vi "test_Open TCP connection using Clear Error node.vi"(8 "error in (no error)":errorcluster, 11 "TestCase in":refnum<class "Ethernet Protocol Tests.lvclass">) -> (0 "error out":errorcluster, 3 "TestCase out":refnum<class "Ethernet Protocol Tests.lvclass">)   [LabVIEW 2019, in "Ethernet Protocol Tests.lvclass"]
uses:
  Ethernet Protocol Tests.lvclass
  TCP/TCP.lvclass
  TCP/TCP.lvclass/TCP.ctl
  Constants.vi
  <vilib>/addons/_JKI Toolkits/VI Tester/TestCase.llb/TestCase.lvclass
  C:/Program Files (x86)/National Instruments/LabVIEW 2019/vi.lib/addons/_JKI Toolkits/VI Tester/TestCase.llb/TestCase.lvclass
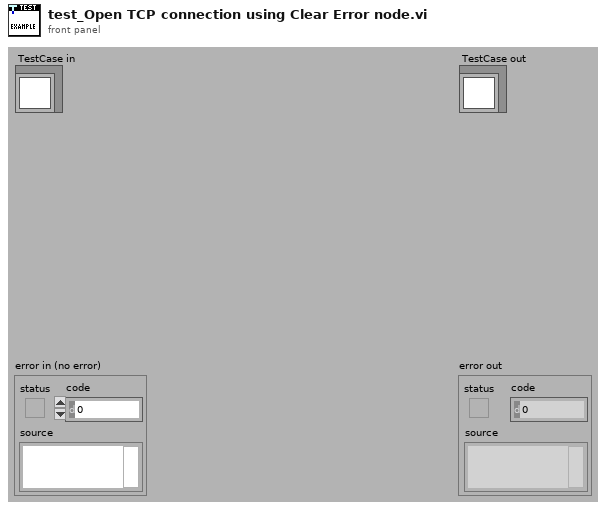
[diagram p1: front panel]
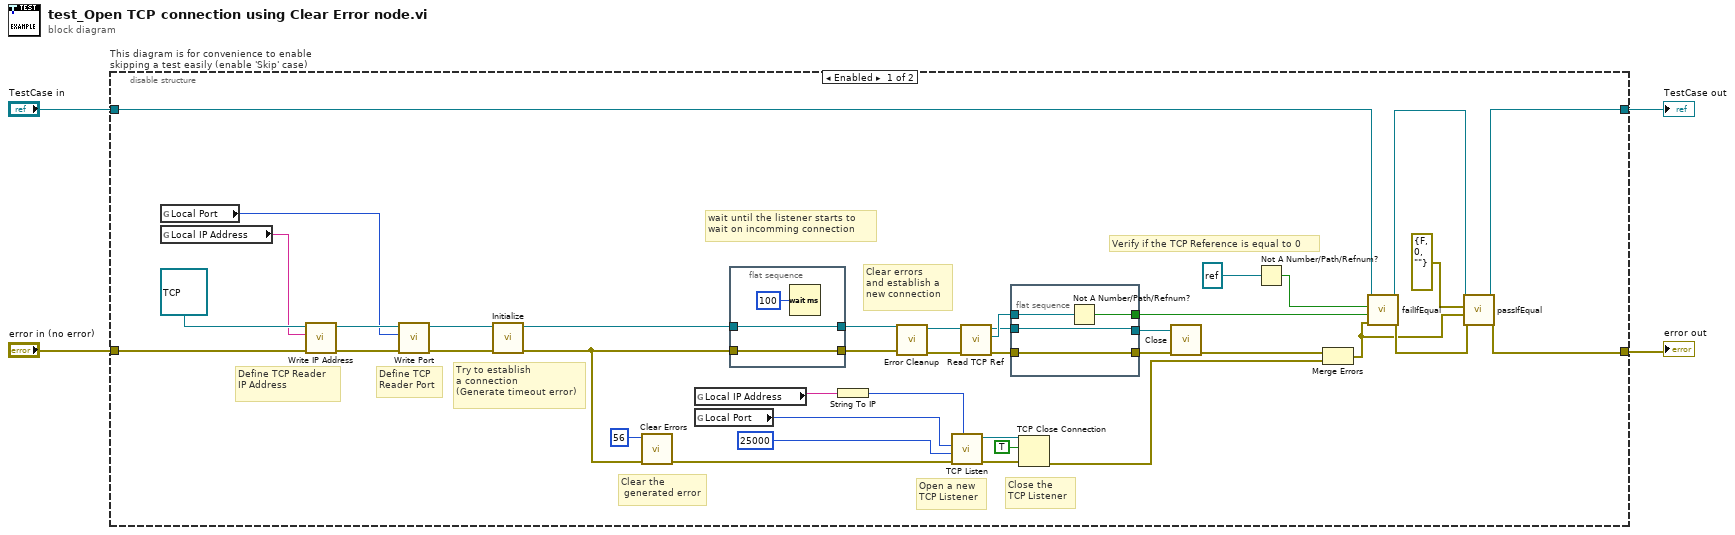
[diagram p0: block diagram]
diagram:
  n1 = disable-structure "This diagram is for convenience to enable skipping a test easily (enable 'Skip' case)" shown="Enabled" {
    disable-tunnel: "TestCase in" -> [w44 w55]
    disable-tunnel: [w12 w53] -> w1
    disable-tunnel: [w11 w54] -> w3
    disable-tunnel: "error in (no error)" -> [w40 w52]
    frame Enabled {
      # "Verify if the TCP Reference is equal to 0"
      # "Clear the\n generated error"
      # "Close the \nTCP Listener"
      # "Open a new \nTCP Listener"
      # "Clear errors \nand establish a \nnew connection"
      # "Try to establish \na connection\n(Generate timeout error)"
      # "wait until the listener starts to\nwait on incomming connection"
      # "Define TCP \nReader Port"
      # "Define TCP Reader \nIP Address"
      n2 = global read "Constants.vi" "Local Port"() -> (w19:u16)
      n3 = global read "Constants.vi" "Local IP Address"() -> (w20:string)
      n4 = call "Write IP Address.vi"("error in (no error)"=w40, "IP Address"=w20, "Ethernet in"=refnum<class "TCP.lvclass"> refnum ("Protocols.lvlib:TCP.lvclass")) -> ("error out"=w42:errorcluster, "Ethernet out"=w43:refnum<class "TCP.lvclass">)  [unwired: 7 in]
      n5 = call "Write Port.vi"("error in (no error)"=w42, "Port"=w19, "Ethernet in"=w43) -> ("error out"=w39:errorcluster, "Ethernet out"=w38:refnum<class "TCP.lvclass">)  [unwired: 7 in]
      n6 = call-dynamic "Initialize.vi"("error in (no error)"=w39, "Ethernet in"=w38) -> ("error out"=w32:errorcluster, "Ethernet out"=w31:refnum<class "TCP.lvclass">)  [unwired: 8 in]
      n7 = call <vilib>:"Clear Errors.vi"("error in (no error)"=w32, "specific error code to clear (0: all)"=56) -> ("error out"=w33:errorcluster)  [unwired: 4 in, 1 out]
      n8 = global read "Constants.vi" "Local IP Address"() -> (w18:string)
      n9 = global read "Constants.vi" "Local Port"() -> (w17:u16)
      n10 = flat-sequence {
        tunnel: w32 -> [w51]
        tunnel: w31 -> [w50]
        tunnel: [w51] -> w35
        tunnel: [w50] -> w34
        frame #0 {
          n11 = Wait (ms)(milliseconds to wait=u32 100) -> ()  [unwired: 1 out]
        }
      }
      n12 = String To IP(1:w18) -> (0:w37:u32)
      n13 = call-dynamic "Error Cleanup.vi"("error in (no error)"=w35, "Ethernet in"=w34) -> ("error out"=w25:errorcluster, "Ethernet out"=w24:refnum<class "TCP.lvclass">)  [unwired: 8 in]
      n14 = call <vilib>:"TCP Listen.vi"("net address"=w37, "error in (no error)"=w33, "timeout ms (wait forever: -1)"=25000, "port"=w17) -> ("error out"=w29:errorcluster, "connection ID"=w28:refnum<k5>)  [unwired: 3 in, 3 out]
      n15 = call "Read TCP Ref.vi"("error in (no error)"=w25, "Ethernet in"=w24) -> ("error out"=w6:errorcluster, "TCP Ref"=w9:refnum<k5>, "Ethernet out"=w8:refnum<class "TCP.lvclass">)  [unwired: 7 in]
      n16 = flat-sequence {
        tunnel: [w48] -> w10
        tunnel: w9 -> [w47]
        tunnel: w8 -> [w46]
        tunnel: [w46] -> w7
        tunnel: w6 -> [w45]
        tunnel: [w45] -> w5
        frame #0 {
          n17 = Not A Number/Path/Refnum?(number/path/refnum=w47) -> (NaN/Path/Refnum?=w48:bool)
        }
      }
      n18 = TCP Close Connection(connection ID=w28, abort (F)=TRUE, error in (no error)=w29) -> (error out=w26:errorcluster)  [unwired: 1 out]
      n19 = call-dynamic "Close.vi"("error in (no error)"=w5, "Ethernet in"=w7) -> ("error out"=w21:errorcluster)  [unwired: 8 in, 1 out]
      n20 = Not A Number/Path/Refnum?(number/path/refnum=refnum<k5> refnum ("TCP Ref")) -> (NaN/Path/Refnum?=w22:bool)
      n21 = Merge Errors(w21, w26) -> (w13:errorcluster)
      n22 = call-dynamic "failIfEqual.vi"("error in (no error)"=w13, "y"=w10, "x"=w22, "TestCase in"=w44) -> ("error out"=w16:errorcluster, "TestCase out"=w15:refnum<class "Ethernet Protocol Tests.lvclass">)  [unwired: 6 in]
      n23 = call-dynamic "passIfEqual.vi"("error in (no error)"=w16, "y"=w13, "x"=errorcluster {"status"=FALSE, "code"=0, "source"=""} ("error constant"), "TestCase in"=w15) -> ("error out"=w11:errorcluster, "TestCase out"=w12:refnum<class "Ethernet Protocol Tests.lvclass">)  [unwired: 6 in]
    }
    frame Disabled {
      # "skip test result while test is under development"
      n24 = call <vilib>:"skip.vi"("error in (no error)"=w52, "TestCase in"=w55) -> ("error out"=w54:errorcluster, "TestCase out"=w53:refnum<class "Ethernet Protocol Tests.lvclass">)  [unwired: 8 in]
    }
  }
  "error out" <- w3
  "TestCase out" <- w1
